vi "ADIS16448 Loop Update Status.vi"(8 "error in (no error)":errorcluster, 11 "ADIS16448 Status":T1) -> (0 "error out":errorcluster)   [LabVIEW 2019]
uses:
  Typedef/ADIS16448 Status.ctl
  ADIS16448 Globals.vi
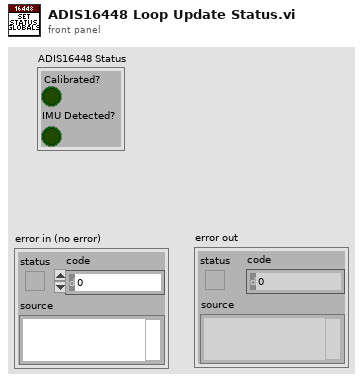
[diagram p1: front panel]
types:
  T1 = typedef "ADIS16448 Status.ctl" = cluster{"Calibrated?":bool, "IMU Detected?":bool}
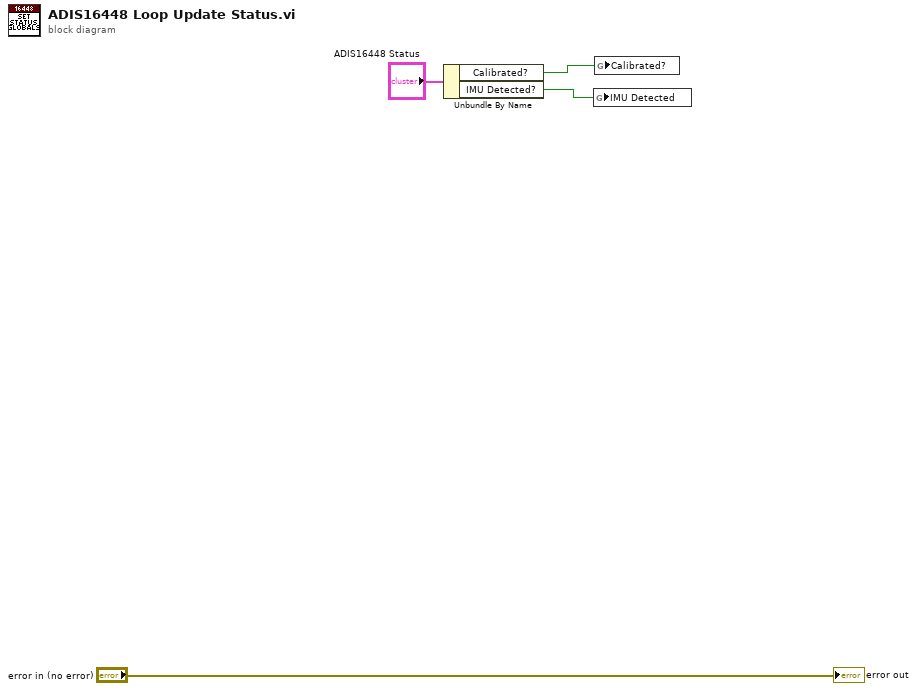
[diagram p0: block diagram]
diagram:
  n1 = Unbundle By Name("ADIS16448 Status") -> ("Calibrated?"=w2:bool, "IMU Detected?"=w1:bool)
  n2 = global write "ADIS16448 Globals.vi" "IMU Detected"(w1) -> ()
  n3 = global write "ADIS16448 Globals.vi" "Calibrated?"(w2) -> ()
  "error out" <- "error in (no error)"
